vi "Cluster Node_Unwired Terminals.vi"(8 "error in":errorcluster, 10 "Named Unbundler Ref":refnum<vi>, 11 "Named Bundler Ref":refnum<vi>) -> (0 "error out":errorcluster, 1 "Unwired Indices For Removal":i32[](array[numeric]), 2 "Unwired Indices":i32[](array[numeric]))   [LabVIEW 2023]
doc: "Returns list of unwired terminals, and a separate list of those the can be removed. The latter will be different if all terminals are unwired, because you cannot remove *all* unwired terminals from the node."
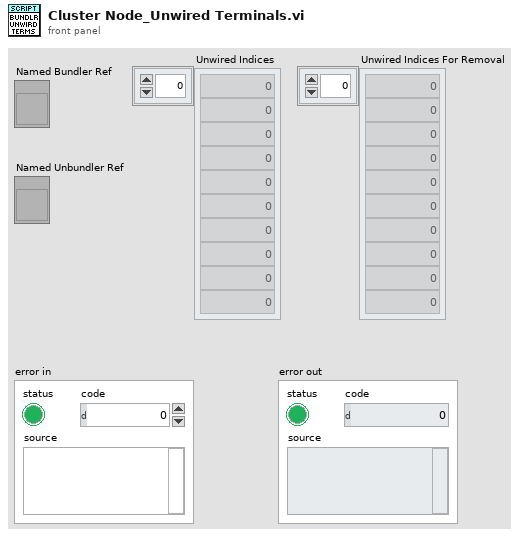
[diagram p1: front panel]
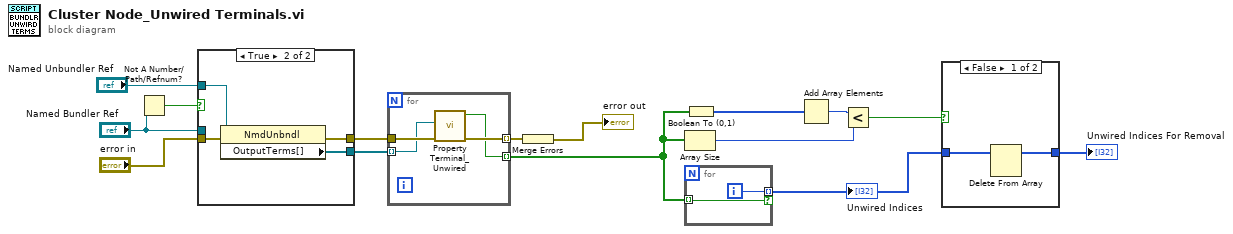
[diagram p0: block diagram]
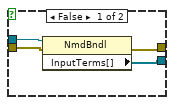
[diagram p2: hidden frame]
diagram:
  n1 = Not A Number/Path/Refnum?(number/path/refnum="Named Bundler Ref") -> (NaN/Path/Refnum?=w3:bool)
  n2 = case shown="True" w3 {
    tunnel: "error in" -> [w19 w23]
    tunnel: [w17 w22] -> w10
    tunnel: [w16 w21] -> w4
    tunnel: "Named Bundler Ref" -> [w18 _]
    tunnel: "Named Unbundler Ref" -> [_ w20]
    frame False {
      n3 = property class="NmdBndl"(reference=w18, error in=w19) -> (error out=w17:errorcluster, "InputTerms[]"=w16:refnum<vi>[])  [unwired: 1 out]
    }
    frame True {
      n4 = property class="NmdUnbndl"(reference=w20, error in=w23) -> (error out=w22:errorcluster, "OutputTerms[]"=w21:refnum<vi>[])  [unwired: 1 out]
    }
  }
  n5 = for {
    tunnel: [w24] -> w9 mode=indexing
    tunnel: w10 -> [w27]
    tunnel: [w26] -> w8 mode=indexing
    tunnel: w4 -> [w25] mode=indexing
    n6 = call "Property Terminal_Unwired.vi"("error in"=w27, "Term Refnum"=w25) -> ("error out"=w26:errorcluster, "Unwired"=w24:bool)  [unwired: 7 in, 1 out]
  }
  n7 = Merge Errors(w8) -> (→"error out":errorcluster)
  n8 = Array Size(array=w9) -> (size(s)=w6:i32)
  n9 = for {
    tunnel: w9 -> [w28] mode=indexing
    tunnel: [w29] -> w14 mode=indexing if=w28
    i -> [w29]
  }
  "Unwired Indices" <- w14
  n10 = Boolean To (0,1)(Boolean=w9) -> (0, 1=w15:i16[])
  n11 = Add Array Elements(numeric array=w15) -> (sum=w7:i16)
  n12 = Less?(x=w7, y=w6) -> (x < y?=w5:bool)
  n13 = case shown="False" w5 {
    tunnel: w14 -> [w31 w32]
    tunnel: [w30 w32] -> w13
    frame False {
      n14 = Delete From Array(array=w31) -> (array with subset deleted=w30:i32[])  [unwired: 2 in, 1 out]
    }
    frame True {
    }
  }
  "Unwired Indices For Removal" <- w13
